vi "ObtainAllMessageQues.vi"(8 "error in":errorcluster, 9 "Error Que Name":string="Error", 10 "DAQ Que Name":string="DAQ", 11 "Main Que Name":string="Main") -> (0 "error out":errorcluster, 3 "MessageQues":T1)   [LabVIEW 2018]
doc: "This VI creates and initializes all the message queues for your application. If your application requires more than one message queue, right-click the \"Message Queues\" constant above and select Open Type Def. Add the new Message Queue(s) to the type definition, then initialize them in this VI. \n\nThe que names are/can be used in the error handler loop. It can use the names to provide unique error handling for selected state machine loops.\n\nBolder Software LLC"
uses:
  MultipleMessageQues.ctl
  MessageQue.ctl
  MessageCluster.ctl
  MessageQue.lvlib
panel:
  # "The que names are/can be used\nin the error handler loop. It can\nuse the names to provide unique\nerror handling for selected state\nmachine loops."
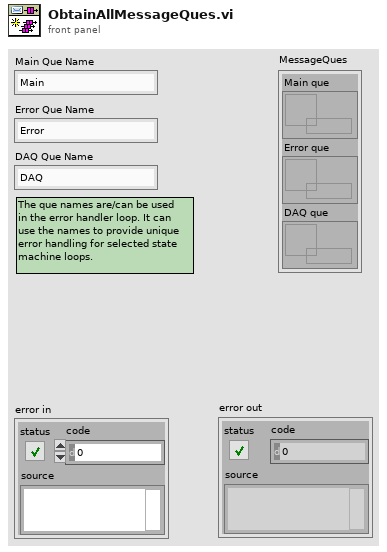
[diagram p1: front panel]
types:
  T1 = typedef "MultipleMessageQues.ctl" = cluster{"Main que":T2, "Error que":T2, "DAQ que":T2}
  T2 = typedef "MessageQue.lvlib/MessageQue.ctl" = refnum<queue>
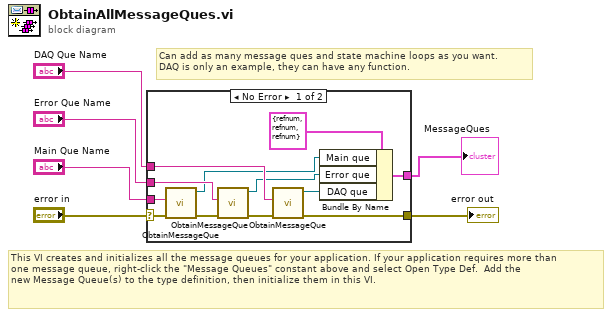
[diagram p0: block diagram]
diagram:
  # "Can add as many message ques and state machine loops as you want. \nDAQ is only an example, they can have any function."
  # "This VI creates and initializes all the message queues for your application. If your application requires more than \none message queue, right-click the \"Message Queues\" constant above and select Open Type Def.  Add the \nnew Message Queue(s) to the type definition, then initialize them in this VI."
  n1 = case shown="No Error" "error in" {
    selector: "error in" -> [w11 w19]
    tunnel: "Main Que Name" -> [w18 _]
    tunnel: [w17 _] -> w3
    tunnel: "Error Que Name" -> [w16 _]
    tunnel: "DAQ Que Name" -> [w15 _]
    tunnel: [w12 w19] -> w5
    frame No Error {
      n2 = call "ObtainMessageQue.vi"("error in"=w11, "Name"=w18) -> ("error out"=w13:errorcluster, "message que out"=w9:T2)  [unwired: 6 in, 2 out]
      n3 = call "ObtainMessageQue.vi"("error in"=w13, "Name"=w16) -> ("error out"=w14:errorcluster, "message que out"=w8:T2)  [unwired: 6 in, 2 out]
      n4 = call "ObtainMessageQue.vi"("error in"=w14, "Name"=w15) -> ("error out"=w12:errorcluster, "message que out"=w7:T2)  [unwired: 6 in, 2 out]
      n5 = Bundle By Name(cluster=T1 {"Main que"=refnum, "Error que"=refnum, "DAQ que"=refnum} ("MessageQues"), "Main que"=w9, "Error que"=w8, "DAQ que"=w7) -> (w17:T1)
    }
    frame Error {
    }
  }
  "error out" <- w5
  "MessageQues" <- w3
